vi "tdtc.vi"(7 "input":dbl, 8 "Tau":dbl=9.49, 9 "Theta":dbl=232.06, 10 "Kss":dbl=1.1, 11 "T0":dbl) -> (2 "output":dbl)   [LabVIEW 2018]
panel:
  # "This takes the first given input as the \nambient tempeerature."
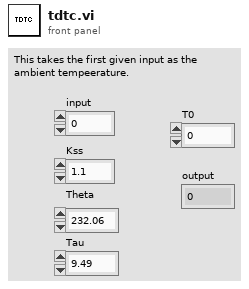
[diagram p1: front panel]
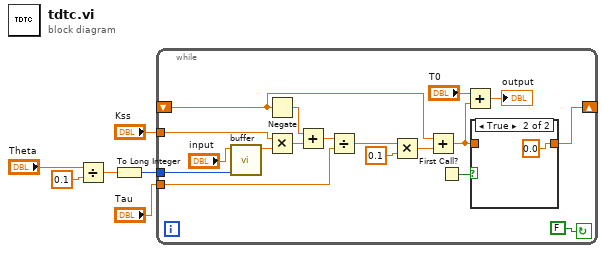
[diagram p0: block diagram]
diagram:
  n1 = Divide(x="Theta", y=0.1) -> (x/y=w4:dbl)
  n2 = To Long Integer(number=w4) -> (32bit integer=w1:i32)
  n3 = while {
    shift-right: [w11] -> _
    shift-left: _ -> [w15]
    tunnel: "Kss" -> [w23]
    tunnel: "Tau" -> [w19]
    tunnel: w1 -> [w14]
    stop <- FALSE continue-if-true
    n4 = call "buffer.vi"("dimension size"=w14, "input"="input") -> ("delayed input"=w13:dbl)  [unwired: 9 in]
    n5 = Negate(x=w15) -> (-x=w22:dbl)
    n6 = Multiply(x=w23, y=w13) -> (x*y=w21:dbl)
    n7 = Add(x=w22, y=w21) -> (x+y=w20:dbl)
    n8 = Divide(x=w20, y=w19) -> (x/y=w18:dbl)
    n9 = Multiply(x=w18, y=0.1) -> (x*y=w16:dbl)
    n10 = Add(x=w15, y=w16) -> (x+y=w7:dbl)
    n11 = First Call?() -> (First Call?: T/F=w12:bool)
    n12 = Add(x="T0", y=w7) -> (x+y=→"output":dbl)
    n13 = case shown="True" w12 {
      tunnel: [w25 0.0] -> w11
      tunnel: w7 -> [w25 _]
      frame False {
      }
      frame True {
      }
    }
  }
